vi "rp_align_objects.vi"(6 "Variant in":variant, 7 "Shift Pressed?":bool, 8 "error in (no error)":errorcluster, 10 "QD Combo Box Ref":refnum<vi>, 11 "QD Launch VI Ref":refnum<vi>) -> (0 "error out":errorcluster, 4 "Variant out":variant)   [LabVIEW 2019]
doc: "Quick align the selected objects using the quick drop combobox text below:\n'X': Align Right Edges & Distribute Vertical Compress\n'XX': Align Left Edges & Distribute Vertical Compress\n'W': Align Top Edges\n'E': Align Vertical Centers\n'S': Align Bottom Edges\n'A': Align Left Edges\n'Q': Align Horizontal Centers\n'D': Align Right Edges\n'WW': Distribute Top Edges\n'QQ': Distribute Vertical Centers\n'SS': Distribute Bottom Edges\n'R': Distribute Vertical Gap\n'F': Distribute Vertical Compress\n'AA': Distribute Left Edges\n'EE': Distribute Horizontal Centers\n'DD': Distribute Right Edges\n'T': Distribute Horizontal Gap\n'G': Distribute Horizontal Compress\n\nExamples:\nAlign Vertical Center = \"q\" + Ctrl-X\nAlign Top + Horizontal Centers = \"w ee\" + Ctrl-X\n\nCreated by: Ryan Pacini\n\nDefault Shortcut - [X]"
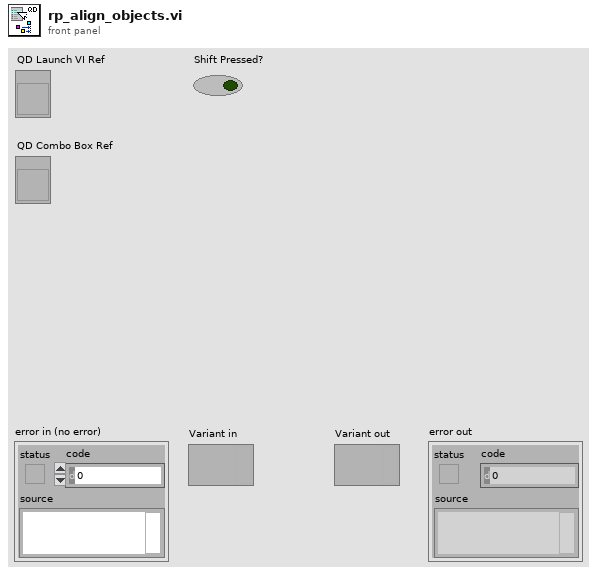
[diagram p1: front panel]
types:
  T1 = enum32{"Top Edges", "Vertical Centers", "Bottom Edges", "Left Edges", "Horizontal Centers", "Right Edges"}
  T2 = enum32{"Top Edges", "Vertical Centers", "Bottom Edges", "Vertical Gap", "Vertical Compress", "Left Edges", "Horizontal Centers", "Right Edges", "Horizontal Gap", "Horizontal Compress"}
  T3 = enum8{"none", "a:Top Edges", "a:Vertical Centers", "a:Bottom Edges", "a:Left Edges", "a:Horizontal Centers", "a:Right Edges", "d:Top Edges", "d:Vertical Centers", "d:Bottom Edges", "d:Vertical Gap", "d:Vertical Compress", "d:Left Edges", "d:Horizontal Centers", "d:Right Edges", "d:Horizontal Gap", "d:Horizontal Compress"}[]
  T4 = cluster{"Label Reference":refnum<vi>, "Visible":bool}
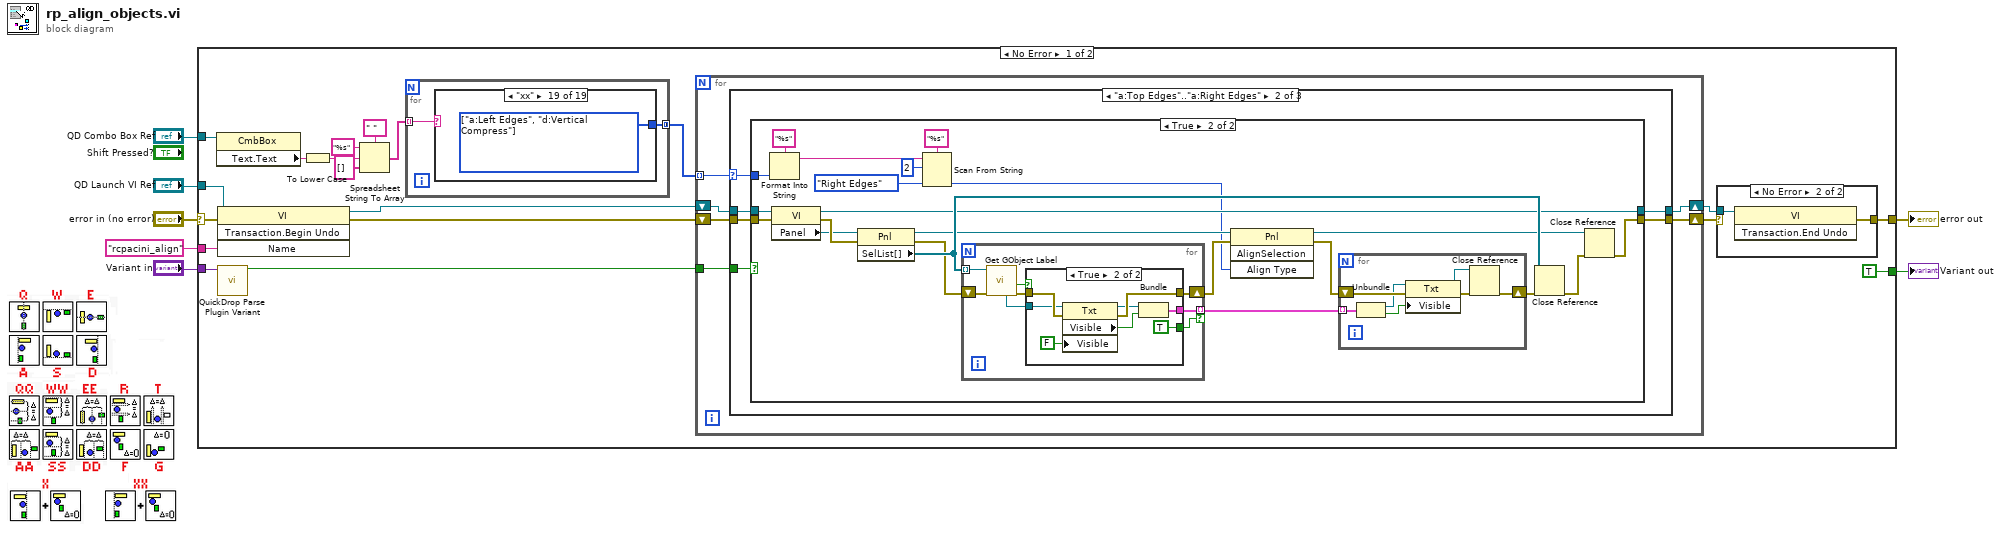
[diagram p0: block diagram]
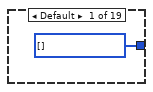
[diagram p2: hidden frame]
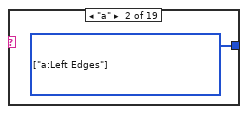
[diagram p3: hidden frame]
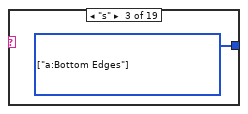
[diagram p4: hidden frame]
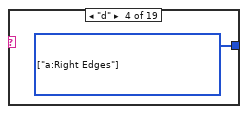
[diagram p5: hidden frame]
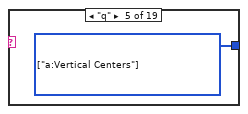
[diagram p6: hidden frame]
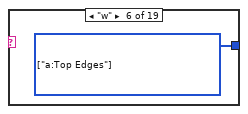
[diagram p7: hidden frame]
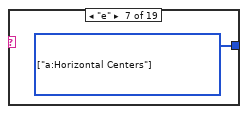
[diagram p8: hidden frame]
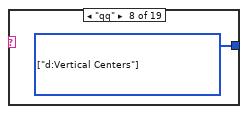
[diagram p9: hidden frame]
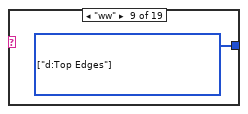
[diagram p10: hidden frame]
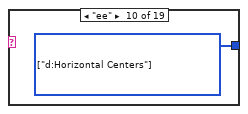
[diagram p11: hidden frame]
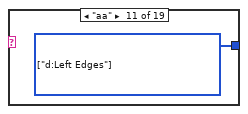
[diagram p12: hidden frame]
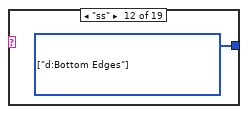
[diagram p13: hidden frame]
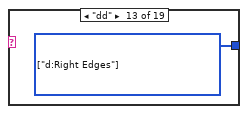
[diagram p14: hidden frame]
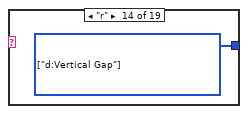
[diagram p15: hidden frame]
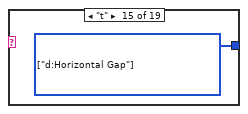
[diagram p16: hidden frame]
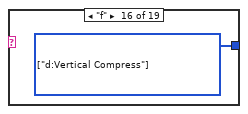
[diagram p17: hidden frame]
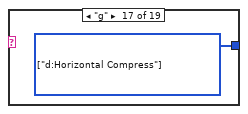
[diagram p18: hidden frame]
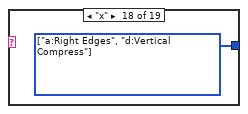
[diagram p19: hidden frame]
diagram:
  n1 = case shown="No Error" "error in (no error)" {
    selector: "error in (no error)" -> [w26 w194]
    tunnel: [w25 w194] -> w2
    tunnel: "QD Launch VI Ref" -> [w16 _]
    tunnel: "rcpacini_align" ("Undo Name") -> [w24 _]
    tunnel: "Variant in" -> [w22 _]
    tunnel: [TRUE _] -> w3
    tunnel: "QD Combo Box Ref" -> [w15 _]
    frame No Error {
      n2 = property class="CmbBox"(reference=w15) -> ("Text.Text"=w14:string)  [unwired: 1 in, 2 out]
      n3 = invoke class="VI" method="Transaction.Begin Undo"(reference=w16, error in=w26, "Name"=w24) -> (reference out=w17:refnum<vi>, error out=w18:errorcluster)  [unwired: 1 in, 2 out]
      n4 = call <vilib>:"QuickDrop Parse Plugin Variant.vi"("QDKS Variant in"=w22) -> ("QD Launch VI Panel?"=w21:bool)  [unwired: 12 in, 2 out]
      n5 = To Lower Case(string=w14) -> (all lower case string=w13:string)
      n6 = Spreadsheet String To Array(delimiter (Tab)=" ", format string="%s", spreadsheet string=w13, array type (2D Dbl)=string[] []) -> (array=w9:string[])
      n7 = for {
        tunnel: w9 -> [w27] mode=indexing
        tunnel: [w28] -> w8 mode=concatenating
        n8 = case shown="\"xx\"" w27 {
          tunnel: [w29 w30 w31 w32 w33 w34 w35 w36 w37 w38 w39 w40 w41 w42 w43 w44 w45 w46 w47] -> w28
          frame Default {
            w29 = T3 [] items=["none", "a:Top Edges", "a:Vertical Centers", "a:Bottom Edges", "a:Left Edges", "a:Horizontal Centers", "a:Right Edges", "d:Top Edges", "d:Vertical Centers", "d:Bottom Edges", "d:Vertical Gap", "d:Vertical Compress", "d:Left Edges", "d:Horizontal Centers", "d:Right Edges", "d:Horizontal Gap", "d:Horizontal Compress"] ("align")
          }
          frame "a" {
            w30 = T3 [enum."a:Left Edges"] items=["none", "a:Top Edges", "a:Vertical Centers", "a:Bottom Edges", "a:Left Edges", "a:Horizontal Centers", "a:Right Edges", "d:Top Edges", "d:Vertical Centers", "d:Bottom Edges", "d:Vertical Gap", "d:Vertical Compress", "d:Left Edges", "d:Horizontal Centers", "d:Right Edges", "d:Horizontal Gap", "d:Horizontal Compress"] ("align")
          }
          frame "s" {
            w31 = T3 [enum."a:Bottom Edges"] items=["none", "a:Top Edges", "a:Vertical Centers", "a:Bottom Edges", "a:Left Edges", "a:Horizontal Centers", "a:Right Edges", "d:Top Edges", "d:Vertical Centers", "d:Bottom Edges", "d:Vertical Gap", "d:Vertical Compress", "d:Left Edges", "d:Horizontal Centers", "d:Right Edges", "d:Horizontal Gap", "d:Horizontal Compress"] ("align")
          }
          frame "d" {
            w32 = T3 [enum."a:Right Edges"] items=["none", "a:Top Edges", "a:Vertical Centers", "a:Bottom Edges", "a:Left Edges", "a:Horizontal Centers", "a:Right Edges", "d:Top Edges", "d:Vertical Centers", "d:Bottom Edges", "d:Vertical Gap", "d:Vertical Compress", "d:Left Edges", "d:Horizontal Centers", "d:Right Edges", "d:Horizontal Gap", "d:Horizontal Compress"] ("align")
          }
          frame "q" {
            w33 = T3 [enum."a:Vertical Centers"] items=["none", "a:Top Edges", "a:Vertical Centers", "a:Bottom Edges", "a:Left Edges", "a:Horizontal Centers", "a:Right Edges", "d:Top Edges", "d:Vertical Centers", "d:Bottom Edges", "d:Vertical Gap", "d:Vertical Compress", "d:Left Edges", "d:Horizontal Centers", "d:Right Edges", "d:Horizontal Gap", "d:Horizontal Compress"] ("align")
          }
          frame "w" {
            w34 = T3 [enum."a:Top Edges"] items=["none", "a:Top Edges", "a:Vertical Centers", "a:Bottom Edges", "a:Left Edges", "a:Horizontal Centers", "a:Right Edges", "d:Top Edges", "d:Vertical Centers", "d:Bottom Edges", "d:Vertical Gap", "d:Vertical Compress", "d:Left Edges", "d:Horizontal Centers", "d:Right Edges", "d:Horizontal Gap", "d:Horizontal Compress"] ("align")
          }
          frame "e" {
            w35 = T3 [enum."a:Horizontal Centers"] items=["none", "a:Top Edges", "a:Vertical Centers", "a:Bottom Edges", "a:Left Edges", "a:Horizontal Centers", "a:Right Edges", "d:Top Edges", "d:Vertical Centers", "d:Bottom Edges", "d:Vertical Gap", "d:Vertical Compress", "d:Left Edges", "d:Horizontal Centers", "d:Right Edges", "d:Horizontal Gap", "d:Horizontal Compress"] ("align")
          }
          frame "qq" {
            w36 = T3 [enum."d:Vertical Centers"] items=["none", "a:Top Edges", "a:Vertical Centers", "a:Bottom Edges", "a:Left Edges", "a:Horizontal Centers", "a:Right Edges", "d:Top Edges", "d:Vertical Centers", "d:Bottom Edges", "d:Vertical Gap", "d:Vertical Compress", "d:Left Edges", "d:Horizontal Centers", "d:Right Edges", "d:Horizontal Gap", "d:Horizontal Compress"] ("align")
          }
          frame "ww" {
            w37 = T3 [enum."d:Top Edges"] items=["none", "a:Top Edges", "a:Vertical Centers", "a:Bottom Edges", "a:Left Edges", "a:Horizontal Centers", "a:Right Edges", "d:Top Edges", "d:Vertical Centers", "d:Bottom Edges", "d:Vertical Gap", "d:Vertical Compress", "d:Left Edges", "d:Horizontal Centers", "d:Right Edges", "d:Horizontal Gap", "d:Horizontal Compress"] ("align")
          }
          frame "ee" {
            w38 = T3 [enum."d:Horizontal Centers"] items=["none", "a:Top Edges", "a:Vertical Centers", "a:Bottom Edges", "a:Left Edges", "a:Horizontal Centers", "a:Right Edges", "d:Top Edges", "d:Vertical Centers", "d:Bottom Edges", "d:Vertical Gap", "d:Vertical Compress", "d:Left Edges", "d:Horizontal Centers", "d:Right Edges", "d:Horizontal Gap", "d:Horizontal Compress"] ("align")
          }
          frame "aa" {
            w39 = T3 [enum."d:Left Edges"] items=["none", "a:Top Edges", "a:Vertical Centers", "a:Bottom Edges", "a:Left Edges", "a:Horizontal Centers", "a:Right Edges", "d:Top Edges", "d:Vertical Centers", "d:Bottom Edges", "d:Vertical Gap", "d:Vertical Compress", "d:Left Edges", "d:Horizontal Centers", "d:Right Edges", "d:Horizontal Gap", "d:Horizontal Compress"] ("align")
          }
          frame "ss" {
            w40 = T3 [enum."d:Bottom Edges"] items=["none", "a:Top Edges", "a:Vertical Centers", "a:Bottom Edges", "a:Left Edges", "a:Horizontal Centers", "a:Right Edges", "d:Top Edges", "d:Vertical Centers", "d:Bottom Edges", "d:Vertical Gap", "d:Vertical Compress", "d:Left Edges", "d:Horizontal Centers", "d:Right Edges", "d:Horizontal Gap", "d:Horizontal Compress"] ("align")
          }
          frame "dd" {
            w41 = T3 [enum."d:Right Edges"] items=["none", "a:Top Edges", "a:Vertical Centers", "a:Bottom Edges", "a:Left Edges", "a:Horizontal Centers", "a:Right Edges", "d:Top Edges", "d:Vertical Centers", "d:Bottom Edges", "d:Vertical Gap", "d:Vertical Compress", "d:Left Edges", "d:Horizontal Centers", "d:Right Edges", "d:Horizontal Gap", "d:Horizontal Compress"] ("align")
          }
          frame "r" {
            w42 = T3 [enum."d:Vertical Gap"] items=["none", "a:Top Edges", "a:Vertical Centers", "a:Bottom Edges", "a:Left Edges", "a:Horizontal Centers", "a:Right Edges", "d:Top Edges", "d:Vertical Centers", "d:Bottom Edges", "d:Vertical Gap", "d:Vertical Compress", "d:Left Edges", "d:Horizontal Centers", "d:Right Edges", "d:Horizontal Gap", "d:Horizontal Compress"] ("align")
          }
          frame "t" {
            w43 = T3 [enum."d:Horizontal Gap"] items=["none", "a:Top Edges", "a:Vertical Centers", "a:Bottom Edges", "a:Left Edges", "a:Horizontal Centers", "a:Right Edges", "d:Top Edges", "d:Vertical Centers", "d:Bottom Edges", "d:Vertical Gap", "d:Vertical Compress", "d:Left Edges", "d:Horizontal Centers", "d:Right Edges", "d:Horizontal Gap", "d:Horizontal Compress"] ("align")
          }
          frame "f" {
            w44 = T3 [enum."d:Vertical Compress"] items=["none", "a:Top Edges", "a:Vertical Centers", "a:Bottom Edges", "a:Left Edges", "a:Horizontal Centers", "a:Right Edges", "d:Top Edges", "d:Vertical Centers", "d:Bottom Edges", "d:Vertical Gap", "d:Vertical Compress", "d:Left Edges", "d:Horizontal Centers", "d:Right Edges", "d:Horizontal Gap", "d:Horizontal Compress"] ("align")
          }
          frame "g" {
            w45 = T3 [enum."d:Horizontal Compress"] items=["none", "a:Top Edges", "a:Vertical Centers", "a:Bottom Edges", "a:Left Edges", "a:Horizontal Centers", "a:Right Edges", "d:Top Edges", "d:Vertical Centers", "d:Bottom Edges", "d:Vertical Gap", "d:Vertical Compress", "d:Left Edges", "d:Horizontal Centers", "d:Right Edges", "d:Horizontal Gap", "d:Horizontal Compress"] ("align")
          }
          frame "x" {
            w46 = T3 [enum."a:Right Edges", enum."d:Vertical Compress"] items=["none", "a:Top Edges", "a:Vertical Centers", "a:Bottom Edges", "a:Left Edges", "a:Horizontal Centers", "a:Right Edges", "d:Top Edges", "d:Vertical Centers", "d:Bottom Edges", "d:Vertical Gap", "d:Vertical Compress", "d:Left Edges", "d:Horizontal Centers", "d:Right Edges", "d:Horizontal Gap", "d:Horizontal Compress"] ("align")
          }
          frame "xx" {
            w47 = T3 [enum."a:Left Edges", enum."d:Vertical Compress"] items=["none", "a:Top Edges", "a:Vertical Centers", "a:Bottom Edges", "a:Left Edges", "a:Horizontal Centers", "a:Right Edges", "d:Top Edges", "d:Vertical Centers", "d:Bottom Edges", "d:Vertical Gap", "d:Vertical Compress", "d:Left Edges", "d:Horizontal Centers", "d:Right Edges", "d:Horizontal Gap", "d:Horizontal Compress"] ("align")
          }
        }
      }
      n9 = for {
        tunnel: w21 -> [w53]
        shift-right: [w51] -> w19
        shift-left: w18 -> [w49]
        shift-right: [w52] -> w20
        shift-left: w17 -> [w50]
        tunnel: w8 -> [w48] mode=indexing
        n10 = case shown="\"a:Top Edges\"..\"a:Right Edges\"" w48 {
          selector: w48 -> [_ w57 w154]
          tunnel: w50 -> [w54 w61 w159]
          tunnel: w53 -> [_ w60 w158]
          tunnel: [w54 w59 w157] -> w52
          tunnel: [w55 w58 w156] -> w51
          tunnel: w49 -> [w55 w56 w155]
          frame "none" {
          }
          frame "a:Top Edges".."a:Right Edges" {
            n11 = case shown="True" w60 {
              tunnel: w56 -> [w78 w124]
              tunnel: w61 -> [w76 w122]
              tunnel: [w77 w123] -> w58
              tunnel: [w73 w119] -> w59
              tunnel: w57 -> [w68 w114]
              frame False {
                n12 = Format Into String(format string="%s", w68) -> (resulting string=w66:string)  [unwired: 2 in, 1 out]
                n13 = property class="VI"(reference=w76, error in=w78) -> (reference out=w73:refnum<vi>, error out=w83:errorcluster, "Diagram"=w74:refnum<vi>)
                n14 = property class="TopLvlDiag"(reference=w74, error in=w83) -> (reference out=w71:refnum<vi>, error out=w80:errorcluster, "SelList[]"=w81:refnum<vi>[])
                n15 = Scan From String(format string="%s", input string=w66, initial scan location=u32 2, default 1=T1."Right Edges" ("Align Type")) -> (output 1=w62:T1)  [unwired: 1 in, 3 out]
                n16 = for {
                  tunnel: w81 -> [w91] mode=indexing
                  shift-right: [w88] -> w72
                  shift-left: w80 -> [w89]
                  tunnel: [w85] -> w75 mode=indexing if=w84
                  n17 = call <vilib>:"Get GObject Label.vi"("error in (no error)"=w89, "GObject"=w91) -> ("error out"=w90:errorcluster, "Object Has Label?"=w87:bool, "Label Reference"=w86:refnum<vi>)  [unwired: 5 in, 2 out]
                  n18 = case shown="True" w87 {
                    tunnel: w90 -> [w92 w100]
                    tunnel: w86 -> [_ w99]
                    tunnel: [w92 w97] -> w88
                    tunnel: [_ w94] -> w85
                    tunnel: [_ TRUE ("Visible")] -> w84
                    frame False {
                    }
                    frame True {
                      n19 = property class="Txt"(reference=w99, error in=w100, "Visible"=FALSE) -> (reference out=w96:refnum<vi>, error out=w97:errorcluster, "Visible"=w95:bool)
                      n20 = Bundle("Label Reference"=w96, "Visible"=w95) -> (w94:T4)  [unwired: 1 in]
                    }
                  }
                }
                n21 = invoke class="TopLvlDiag" method="AlignSelection"(reference=w71, error in=w72, "Align Type"=w62) -> (reference out=w69:refnum<vi>, error out=w70:errorcluster)  [unwired: 1 in, 2 out]
                n22 = for {
                  tunnel: w75 -> [w107] mode=indexing
                  shift-right: [w102] -> w79
                  shift-left: w70 -> [w106]
                  n23 = Unbundle(w107) -> ("Label Reference"=w105:refnum<vi>, "Visible"=w104:bool)
                  n24 = property class="Txt"(reference=w105, error in=w106, "Visible"=w104) -> (reference out=w101:refnum<vi>, error out=w103:errorcluster)
                  n25 = Close Reference(reference=w101, error in (no error)=w103) -> (error out=w102:errorcluster)
                }
                n26 = Close Reference(reference=w81, error in (no error)=w79) -> (error out=w82:errorcluster)
                n27 = Close Reference(reference=w69, error in (no error)=w82) -> (error out=w77:errorcluster)
              }
              frame True {
                n28 = Format Into String(format string="%s", w114) -> (resulting string=w112:string)  [unwired: 2 in, 1 out]
                n29 = property class="VI"(reference=w122, error in=w124) -> (reference out=w119:refnum<vi>, error out=w129:errorcluster, "Panel"=w120:refnum<vi>)
                n30 = property class="Pnl"(reference=w120, error in=w129) -> (reference out=w117:refnum<vi>, error out=w126:errorcluster, "SelList[]"=w127:refnum<vi>[])
                n31 = Scan From String(format string="%s", input string=w112, initial scan location=u32 2, default 1=T1."Right Edges" ("Align Type")) -> (output 1=w108:T1)  [unwired: 1 in, 3 out]
                n32 = for {
                  tunnel: w127 -> [w137] mode=indexing
                  shift-right: [w134] -> w118
                  shift-left: w126 -> [w135]
                  tunnel: [w131] -> w121 mode=indexing if=w130
                  n33 = call <vilib>:"Get GObject Label.vi"("error in (no error)"=w135, "GObject"=w137) -> ("error out"=w136:errorcluster, "Object Has Label?"=w133:bool, "Label Reference"=w132:refnum<vi>)  [unwired: 5 in, 2 out]
                  n34 = case shown="True" w133 {
                    tunnel: w136 -> [w138 w146]
                    tunnel: w132 -> [_ w145]
                    tunnel: [w138 w143] -> w134
                    tunnel: [_ w140] -> w131
                    tunnel: [_ TRUE ("Visible")] -> w130
                    frame False {
                    }
                    frame True {
                      n35 = property class="Txt"(reference=w145, error in=w146, "Visible"=FALSE) -> (reference out=w142:refnum<vi>, error out=w143:errorcluster, "Visible"=w141:bool)
                      n36 = Bundle("Label Reference"=w142, "Visible"=w141) -> (w140:T4)  [unwired: 1 in]
                    }
                  }
                }
                n37 = invoke class="Pnl" method="AlignSelection"(reference=w117, error in=w118, "Align Type"=w108) -> (reference out=w115:refnum<vi>, error out=w116:errorcluster)  [unwired: 1 in, 2 out]
                n38 = for {
                  tunnel: w121 -> [w153] mode=indexing
                  shift-right: [w148] -> w125
                  shift-left: w116 -> [w152]
                  n39 = Unbundle(w153) -> ("Label Reference"=w151:refnum<vi>, "Visible"=w150:bool)
                  n40 = property class="Txt"(reference=w151, error in=w152, "Visible"=w150) -> (reference out=w147:refnum<vi>, error out=w149:errorcluster)
                  n41 = Close Reference(reference=w147, error in (no error)=w149) -> (error out=w148:errorcluster)
                }
                n42 = Close Reference(reference=w127, error in (no error)=w125) -> (error out=w128:errorcluster)
                n43 = Close Reference(reference=w115, error in (no error)=w128) -> (error out=w123:errorcluster)
              }
            }
          }
          frame "d:Top Edges".."d:Horizontal Compress" {
            # "include label/captions when compressing"
            n44 = case shown="False" w158 {
              tunnel: w155 -> [w174 w189]
              tunnel: w159 -> [w172 w187]
              tunnel: [w173 w188] -> w156
              tunnel: [w171 w186] -> w157
              tunnel: w154 -> [w162 w177]
              frame True {
                n45 = Format Into String(format string="%s", w162) -> (resulting string=w165:string)  [unwired: 2 in, 1 out]
                n46 = property class="VI"(reference=w172, error in=w174) -> (reference out=w171:refnum<vi>, error out=w167:errorcluster, "Panel"=w168:refnum<vi>)
                n47 = Scan From String(format string="%s", input string=w165, initial scan location=u32 2, default 1=T2."Vertical Compress" ("DistributeType")) -> (output 1=w160:T2)  [unwired: 1 in, 3 out]
                n48 = invoke class="Pnl" method="DistributeSelection"(reference=w168, error in=w167, "DistributeType"=w160) -> (reference out=w170:refnum<vi>, error out=w169:errorcluster)  [unwired: 1 in, 2 out]
                n49 = Close Reference(reference=w170, error in (no error)=w169) -> (error out=w173:errorcluster)
              }
              frame False {
                n50 = Format Into String(format string="%s", w177) -> (resulting string=w180:string)  [unwired: 2 in, 1 out]
                n51 = property class="VI"(reference=w187, error in=w189) -> (reference out=w186:refnum<vi>, error out=w182:errorcluster, "Diagram"=w183:refnum<vi>)
                n52 = Scan From String(format string="%s", input string=w180, initial scan location=u32 2, default 1=T2."Vertical Compress" ("DistributeType")) -> (output 1=w175:T2)  [unwired: 1 in, 3 out]
                n53 = invoke class="TopLvlDiag" method="DistributeSelection"(reference=w183, error in=w182, "DistributeType"=w175) -> (reference out=w185:refnum<vi>, error out=w184:errorcluster)  [unwired: 1 in, 2 out]
                n54 = Close Reference(reference=w185, error in (no error)=w184) -> (error out=w188:errorcluster)
              }
            }
          }
        }
      }
      n55 = case shown="No Error" w19 {
        tunnel: w20 -> [w190 w192]
        tunnel: [w191 w193] -> w25
        frame Error {
          n56 = invoke class="VI" method="Transaction.Fail"(reference=w190) -> (error out=w191:errorcluster)  [unwired: 2 in, 2 out]
        }
        frame No Error {
          n57 = invoke class="VI" method="Transaction.End Undo"(reference=w192) -> (error out=w193:errorcluster)  [unwired: 2 in, 2 out]
        }
      }
    }
    frame Error {
    }
  }
  "error out" <- w2
  "Variant out" <- w3
